vi "CopyAssetNodePropsToDevice.vi"(9 "KeyValues":T1[](array[typedef]), 10 "AssetNodes":T3[](array[typedef]), 11 "DeviceModel in":T14) -> (3 "DeviceModel out":T14)   [LabVIEW 2017, in "ServerComm.lvlib"]
uses:
  <vilib>/addons/InsightCM/Devices/Shared/Common/ServerComm/ServerComm.lvlib
  <vilib>/addons/InsightCM/MessageBus/Base/controls/R2_DeviceModel.ctl
  <vilib>/addons/InsightCM/MessageBus/Base/controls/R2_Device.ctl
  <vilib>/addons/InsightCM/MessageBus/Base/controls/KeyValuePair.ctl
  <vilib>/addons/InsightCM/MessageBus/Base/controls/DeviceState.ctl
  <vilib>/addons/InsightCM/MessageBus/Base/controls/R2_DataGroup.ctl
  <vilib>/addons/InsightCM/MessageBus/Base/controls/OperatingState.ctl
  <vilib>/addons/InsightCM/MessageBus/Base/controls/Trigger.ctl
  <vilib>/addons/InsightCM/MessageBus/Base/controls/Condition.ctl
  <vilib>/addons/InsightCM/MessageBus/Base/controls/BurstModeTrigger.ctl
  <vilib>/addons/InsightCM/MessageBus/Base/controls/DeviceSensorGroup.ctl
  <vilib>/addons/InsightCM/MessageBus/Base/controls/WirelessEndpoint.ctl
  <vilib>/addons/InsightCM/MessageBus/Base/controls/WirelessChannel.ctl
  <vilib>/addons/InsightCM/MessageBus/Base/controls/R2_Channel.ctl
  <vilib>/addons/InsightCM/MessageBus/Base/controls/Metric.ctl
  <vilib>/addons/InsightCM/MessageBus/Base/controls/Tag.ctl
  <vilib>/addons/InsightCM/MessageBus/Base/controls/AssetNode.ctl
  <vilib>/addons/InsightCM/MessageBus/Base/controls/AssetState.ctl
  <vilib>/addons/InsightCM/MessageBus/Base/controls/AssetNodeSensorGroup.ctl
  <vilib>/addons/InsightCM/MessageBus/Base/controls/TrendAlarmRule.ctl
  <vilib>/addons/InsightCM/MessageBus/Base/controls/TrendAlarmLevel.ctl
  <vilib>/addons/InsightCM/MessageBus/Base/controls/AlarmAction.ctl
  <vilib>/addons/InsightCM/MessageBus/Base/controls/AssetNodeReference.ctl
  <vilib>/addons/InsightCM/MessageBus/Base/controls/SectionKeyValues.ctl
  <vilib>/addons/InsightCM/Utilities/DeviceModelHelpers/DeviceModelHelpers.lvlib
  <vilib>/addons/InsightCM/Utilities/PropertyHelpers/PropertyHelpers.lvlib
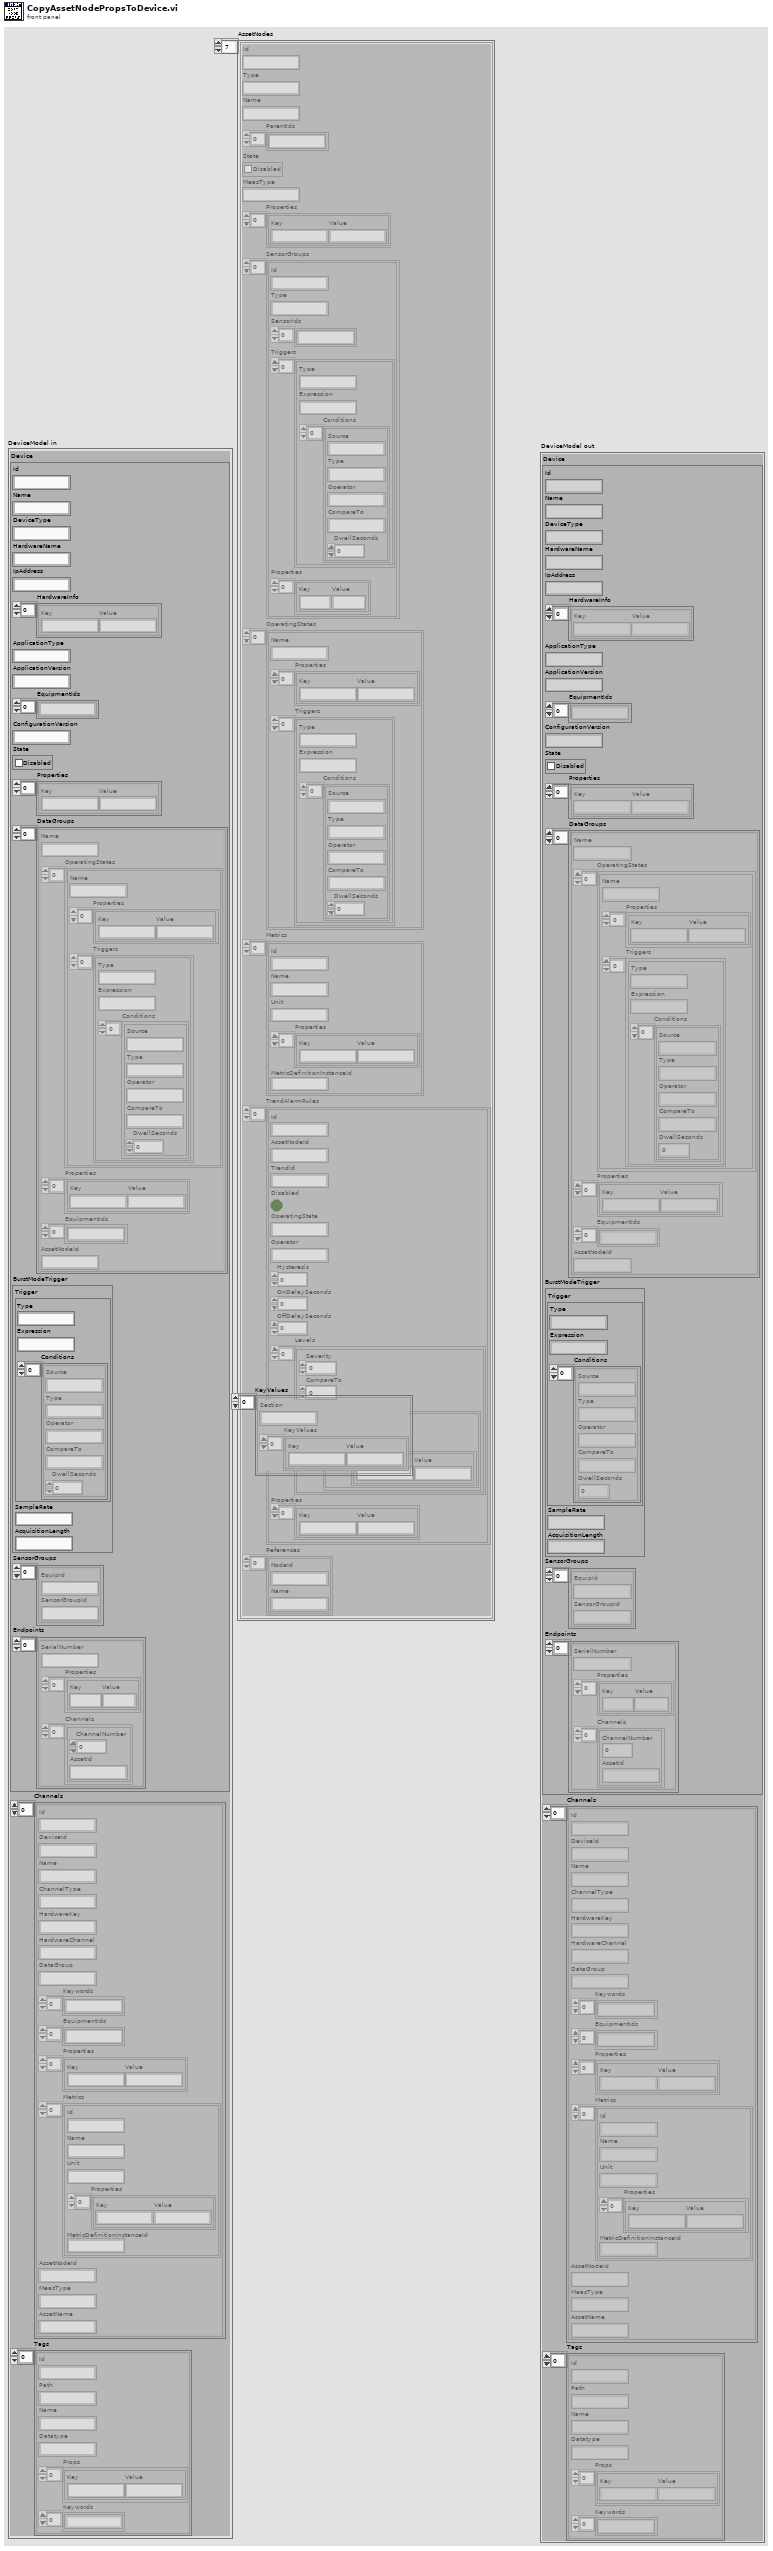
[diagram p1: front panel]
types:
  T1 = typedef "SectionKeyValues.ctl" = cluster{"Section":string, "KeyValues":T2[]}
  T2 = typedef "KeyValuePair.ctl" = cluster{"Key":string, "Value":string}
  T3 = typedef "AssetNode.ctl" = cluster{"Id":string, "Type":string, "Name":string, "ParentIds":string[], "State":T4, "MeasType":string, "Properties":T2[], "SensorGroups":T5[], "OperatingStates":T8[], "Metrics":T9[], "TrendAlarmRules":T10[], "References":T13[]}
  T4 = typedef "AssetState.ctl" = cluster{"Disabled":bool}
  T5 = typedef "AssetNodeSensorGroup.ctl" = cluster{"Id":string, "Type":string, "SensorIds":string[], "Triggers":T6[], "Properties":T2[]}
  T6 = typedef "Trigger.ctl" = cluster{"Type":string, "Expression":string, "Conditions":T7[]}
  T7 = typedef "Condition.ctl" = cluster{"Source":string, "Type":string, "Operator":string, "CompareTo":string, "DwellSeconds":dbl}
  T8 = typedef "OperatingState.ctl" = cluster{"Name":string, "Properties":T2[], "Triggers":T6[]}
  T9 = typedef "Metric.ctl" = cluster{"Id":string, "Name":string, "Unit":string, "Properties":T2[], "MetricDefinitionInstanceId":string}
  T10 = typedef "TrendAlarmRule.ctl" = cluster{"Id":string, "AssetNodeId":string, "TrendId":string, "Disabled":bool, "OperatingState":string, "Operator":string, "Hysteresis":dbl, "OnDelaySeconds":dbl, "OffDelaySeconds":dbl, "Levels":T11[], "Properties":T2[]}
  T11 = typedef "TrendAlarmLevel.ctl" = cluster{"Severity":i32, "CompareTo":dbl, "Actions":T12[]}
  T12 = typedef "AlarmAction.ctl" = cluster{"Type":string, "Props":T2[]}
  T13 = typedef "AssetNodeReference.ctl" = cluster{"NodeId":string, "Name":string}
  T14 = typedef "R2_DeviceModel.ctl" = cluster{"Device":T15, "Channels":T22[], "Tags":T23[]}
  T15 = typedef "R2_Device.ctl" = cluster{"Id":string, "Name":string, "DeviceType":string, "HardwareName":string, "IpAddress":string, "HardwareInfo":T2[], "ApplicationType":string, "ApplicationVersion":string, "EquipmentIds":string[], "ConfigurationVersion":string, "State":T16, "Properties":T2[], "DataGroups":T17[], "BurstModeTrigger":T18, "SensorGroups":T19[], "Endpoints":T20[]}
  T16 = typedef "DeviceState.ctl" = cluster{"Disabled":bool}
  T17 = typedef "R2_DataGroup.ctl" = cluster{"Name":string, "OperatingStates":T8[], "Properties":T2[], "EquipmentIds":string[], "AssetNodeId":string}
  T18 = typedef "BurstModeTrigger.ctl" = cluster{"Trigger":T6, "SampleRate":string, "AcquisitionLength":string}
  T19 = typedef "DeviceSensorGroup.ctl" = cluster{"EquipId":string, "SensorGroupId":string}
  T20 = typedef "WirelessEndpoint.ctl" = cluster{"SerialNumber":string, "Properties":T2[], "Channels":T21[]}
  T21 = typedef "WirelessChannel.ctl" = cluster{"ChannelNumber":i32, "AssetId":string}
  T22 = typedef "R2_Channel.ctl" = cluster{"Id":string, "DeviceId":string, "Name":string, "ChannelType":string, "HardwareKey":string, "HardwareChannel":string, "DataGroup":string, "Keywords":string[], "EquipmentIds":string[], "Properties":T2[], "Metrics":T9[], "AssetNodeId":string, "MeasType":string, "AssetName":string}
  T23 = typedef "Tag.ctl" = cluster{"Id":string, "Path":string, "Name":string, "Datatype":string, "Props":T2[], "Keywords":string[]}
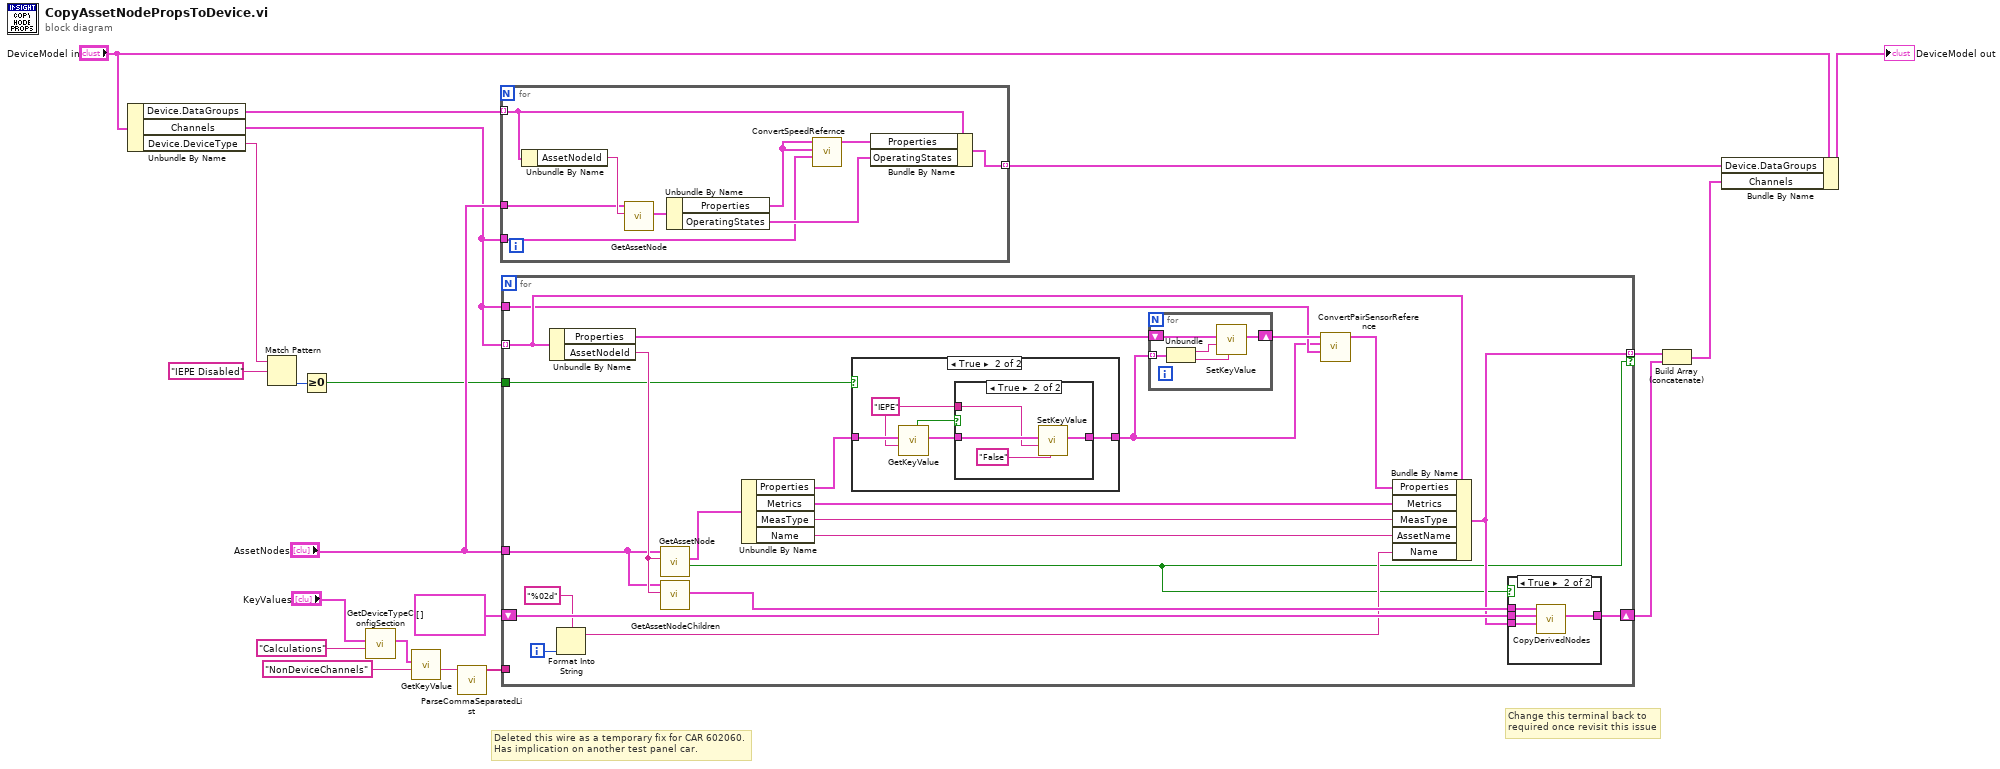
[diagram p0: block diagram]
diagram:
  # "Deleted this wire as a temporary fix for CAR 602060.\nHas implication on another test panel car."
  # "Change this terminal back to\nrequired once revisit this issue"
  n1 = Unbundle By Name("DeviceModel in") -> ("Device.DataGroups"=w17:T17[], "Channels"=w11:T22[], "Device.DeviceType"=w3:string)
  n2 = Match Pattern(string=w3, regular expression="IEPE Disabled") -> (offset past match=w4:i32)  [unwired: 1 in, 3 out]
  n3 = Greater Or Equal To 0?(x=w4) -> (x >= 0?=w1:bool)
  n4 = call <vilib>:"GetDeviceTypeConfigSection.vi"("key"="Calculations", "key values"="KeyValues") -> ("key value pairs out"=w8:T2[])  [unwired: 8 in, 1 out]
  n5 = call <vilib>:"GetKeyValue.vi"("key"="NonDeviceChannels", "key value pairs"=w8) -> ("value"=w6:string)  [unwired: 7 in, 2 out]
  n6 = call <vilib>:"ParseCommaSeparatedList.vi"("List"=w6) -> ("Array"=w5:string[])  [unwired: 10 in]
  n7 = for {
    tunnel: w17 -> [w29] mode=indexing
    tunnel: [w23] -> w16 mode=indexing
    tunnel: w11 -> [w22]
    tunnel: "AssetNodes" -> [w24]
    n8 = Unbundle By Name(w29) -> ("AssetNodeId"=w26:string)
    n9 = call <vilib>:"GetAssetNode.vi"("node id"=w26, "nodes in"=w24) -> ("AssetNode"=w25:T3)  [unwired: 7 in, 2 out]
    n10 = Unbundle By Name(w25) -> ("Properties"=w21:T2[], "OperatingStates"=w28:T8[])
    n11 = call <vilib>:"ConvertSpeedRefernce.vi"("channels"=w22, "node properties"=w21, "dg properties in"=w21) -> ("dg properties out"=w27:T2[])  [unwired: 8 in]
    n12 = Bundle By Name(cluster=w29, "Properties"=w27, "OperatingStates"=w28) -> (w23:T17)
  }
  n13 = for {
    tunnel: w11 -> [w41] mode=indexing
    tunnel: [w40] -> w12 mode=indexing if=w30
    tunnel: "AssetNodes" -> [w46]
    shift-right: [w44] -> w14
    shift-left: T22[] [] ("channels out") -> [w43]
    tunnel: w11 -> [w37]
    tunnel: w5 -> [_]
    tunnel: w1 -> [w33]
    i -> [w36]
    n14 = Unbundle By Name(w41) -> ("Properties"=w51:T2[], "AssetNodeId"=w47:string)
    n15 = Format Into String(format string="%02d", w36) -> (resulting string=w34:string)  [unwired: 2 in, 1 out]
    n16 = call <vilib>:"GetAssetNode.vi"("node id"=w47, "nodes in"=w46) -> ("found"=w30:bool, "AssetNode"=w48:T3)  [unwired: 7 in, 1 out]
    n17 = call <vilib>:"GetAssetNodeChildren.vi"("node id"=w47, "nodes in"=w46) -> ("Children"=w45:T3[])  [unwired: 8 in, 1 out]
    n18 = Unbundle By Name(w48) -> ("Properties"=w32:T2[], "Metrics"=w50:T9[], "MeasType"=w49:string, "Name"=w42:string)
    n19 = case shown="True" w33 {
      tunnel: [w52 w55] -> w31
      tunnel: w32 -> [w52 w57]
      frame False {
      }
      frame True {
        w53 = "IEPE" ("key")
        n20 = call <vilib>:"GetKeyValue.vi"("key"=w53, "key value pairs"=w57) -> ("key value pairs out"=w54:T2[], "found"=w56:bool)  [unwired: 7 in, 1 out]
        n21 = case shown="True" w56 {
          tunnel: [w58 w61] -> w55
          tunnel: w54 -> [w58 w62]
          tunnel: w53 -> [_ w60]
          frame False {
          }
          frame True {
            n22 = call <vilib>:"SetKeyValue.vi"("value"="False", "key"=w60, "key value pairs"=w62) -> ("key value pairs out"=w61:T2[])  [unwired: 8 in]
          }
        }
      }
    }
    n23 = for {
      shift-right: [w70] -> w39
      shift-left: w51 -> [w71]
      tunnel: w31 -> [w72] mode=indexing
      n24 = Unbundle(w72) -> ("Key"=w69:string, "Value"=w68:string)
      n25 = call <vilib>:"SetKeyValue.vi"("value"=w68, "key"=w69, "key value pairs"=w71) -> ("key value pairs out"=w70:T2[])  [unwired: 8 in]
    }
    n26 = call <vilib>:"ConvertPairSensorReference.vi"("channels"=w37, "node properties"=w31, "chan properties in"=w39) -> ("chan properties out"=w38:T2[])  [unwired: 8 in]
    n27 = Bundle By Name(cluster=w41, "Properties"=w38, "Metrics"=w50, "MeasType"=w49, "AssetName"=w42, "Name"=w34) -> (w40:T22)
    n28 = case shown="True" w30 {
      tunnel: w45 -> [_ w67]
      tunnel: [w63 w66] -> w44
      tunnel: w43 -> [w63 w65]
      tunnel: w40 -> [_ w64]
      frame False {
      }
      frame True {
        n29 = call <vilib>:"CopyDerivedNodes.vi"("parent channel"=w64, "channels in"=w65, "child nodes"=w67) -> ("channels out"=w66:T22[])  [unwired: 8 in]
      }
    }
  }
  n30 = Build Array (concatenate)(w12, w14) -> (w13:T22[])
  n31 = Bundle By Name(cluster="DeviceModel in", "Device.DataGroups"=w16, "Channels"=w13) -> (→"DeviceModel out":T14)
